vi "Teleop.vi"(10 "Match Info":T1={"Autonomous Elapsed Seconds"=0.0, "TeleOp Elapsed Seconds"=0.0, "Disabled Elapsed Seconds"=0.0, "Visited Autonomous"=FALSE, "Visited TeleOp"=FALSE, "Visited Disabled"=FALSE, "Autonomous Settings"={"Autonomous Style"=enum."Independent", "VI Refnum"=refnum}}, 11 "Call Context":T2) -> ()   [LabVIEW 2023]
doc: "This VI is called for each TeleOp packet received from the DS where the robot is not disabled. It is often used to read from the joysticks and update I/O or to update setpoints for timed control loops. It should complete and return within 20 milliseconds or it may miss DS packets."
uses:
  <vilib>/Rock Robotics/WPI/DriverStation/WPI_DriverStationDerivedRobotMode.ctl
  <vilib>/Rock Robotics/WPI/DriverStation/WPI_DriverStationMatch Info.ctl
  <vilib>/Rock Robotics/WPI/Utilities/WPI_GetSetVariantRefNum.vi
  <vilib>/Rock Robotics/Network Tables/NT Write Boolean Array.vi
  <vilib>/Rock Robotics/Network Tables/NT Write Numeric Array.vi
  <vilib>/Rock Robotics/Network Tables/NT Read Boolean.vi
  <vilib>/Rock Robotics/Network Tables/NT Read Number.vi
  <vilib>/Rock Robotics/WPI/RobotDrive/WPI_RobotDriveMecanumDrive_Cartesian.vi
panel:
  out "Sample Slider 0":dbl(slide) scale=0.0..5.0
  out "Sample Boolean 1":bool
  out "Sample Boolean 0":bool
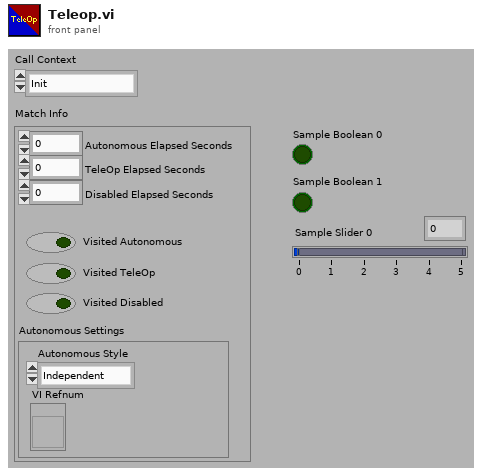
[diagram p1: front panel]
types:
  T1 = typedef "WPI_DriverStationMatch Info.ctl" = cluster{"Autonomous Elapsed Seconds":dbl, "TeleOp Elapsed Seconds":dbl, "Disabled Elapsed Seconds":dbl, "Visited Autonomous":bool, "Visited TeleOp":bool, "Visited Disabled":bool, "Autonomous Settings":cluster{"Autonomous Style":enum16{"Iterative", "Independent"}, "VI Refnum":refnum<vi>}}
  T2 = typedef "WPI_DriverStationDerivedRobotMode.ctl" = enum16{"Init", "Execute", "Stop"}
  T3 = typedef "WPI_JoystickDevRef.ctl" = cluster{"Device":T4}
  T4 = typedef "WPI_JoystickDeviceEnum.ctl" = enum16{"USB 0", "USB 1", "USB 2", "USB 3", "USB 4", "USB 5"}
  T5 = typedef "WPI_MotorControlDeviceRef.ctl" = cluster{"DeviceStatus":errorcluster, "Type":T6, "PWM":cluster{"PWM Channel":T7, "DeadBand":T8}, "CAN":cluster{"Device Number":u8, "SetOutput VI Ref":variant, "GetOutput VI Ref":variant, "Enable VI Ref":variant, "Disable VI Ref":variant, "Data":variant}, "Invert":bool, "DIO PWM":cluster{"PWM \"Enable\" Channel":T7, "DIOChannel":T9, "PWM Rate":dbl}}
  T6 = typedef "WPI_MotorControlType.ctl" = enum16{"PWM", "CAN", "DIO PWM"}
  T7 = typedef "FPGA_DIOPWMChannel.ctl" = enum8{"PWM 0", "PWM 1", "PWM 2", "PWM 3", "PWM 4", "PWM 5", "PWM 6", "PWM 7", "PWM 8", "PWM 9", "PWM MXP 0", "PWM MXP 1", "PWM MXP 2", "PWM MXP 3", "PWM MXP 4", "PWM MXP 5", "PWM MXP 6", "PWM MXP 7", "PWM MXP 8", "PWM MXP 9", "Invalid"}
  T8 = typedef "WPI_PWMDeadband.ctl" = cluster{"Name":string, "maxPositivePwm":i32, "minPositivePwm":i32, "centerPwm":i32, "maxNegativePwm":i32, "minNegativePwm":i32, "angularRange":u16}
  T9 = typedef "FPGA_DIOChannel.ctl" = enum8{"DIO 0", "DIO 1", "DIO 2", "DIO 3", "DIO 4", "DIO 5", "DIO 6", "DIO 7", "DIO 8", "DIO 9", "DIO MXP 0", "DIO MXP 1", "DIO MXP 2", "DIO MXP 3", "DIO MXP 4", "DIO MXP 5", "DIO MXP 6", "DIO MXP 7", "DIO MXP 8", "DIO MXP 9", "DIO MXP 10", "DIO MXP 11", "DIO MXP 12", "DIO MXP 13", "DIO MXP 14", "DIO MXP 15", "SPI Port CS1", "SPI Port CS2", "SPI Port CS3", "SPI Port MISO", "SPI Port MOSI", "Invalid"}
  T10 = typedef "WPI_DigitalInputDevRef.ctl" = cluster{"DevStatus":errorcluster, "DIO Channel":T9}
  T11 = typedef "WPI_RobotDriveDevRef.ctl" = cluster{"DevStatus":errorcluster, "Motors[]":T5[], "Square Inputs":bool, "Max Output":dbl}
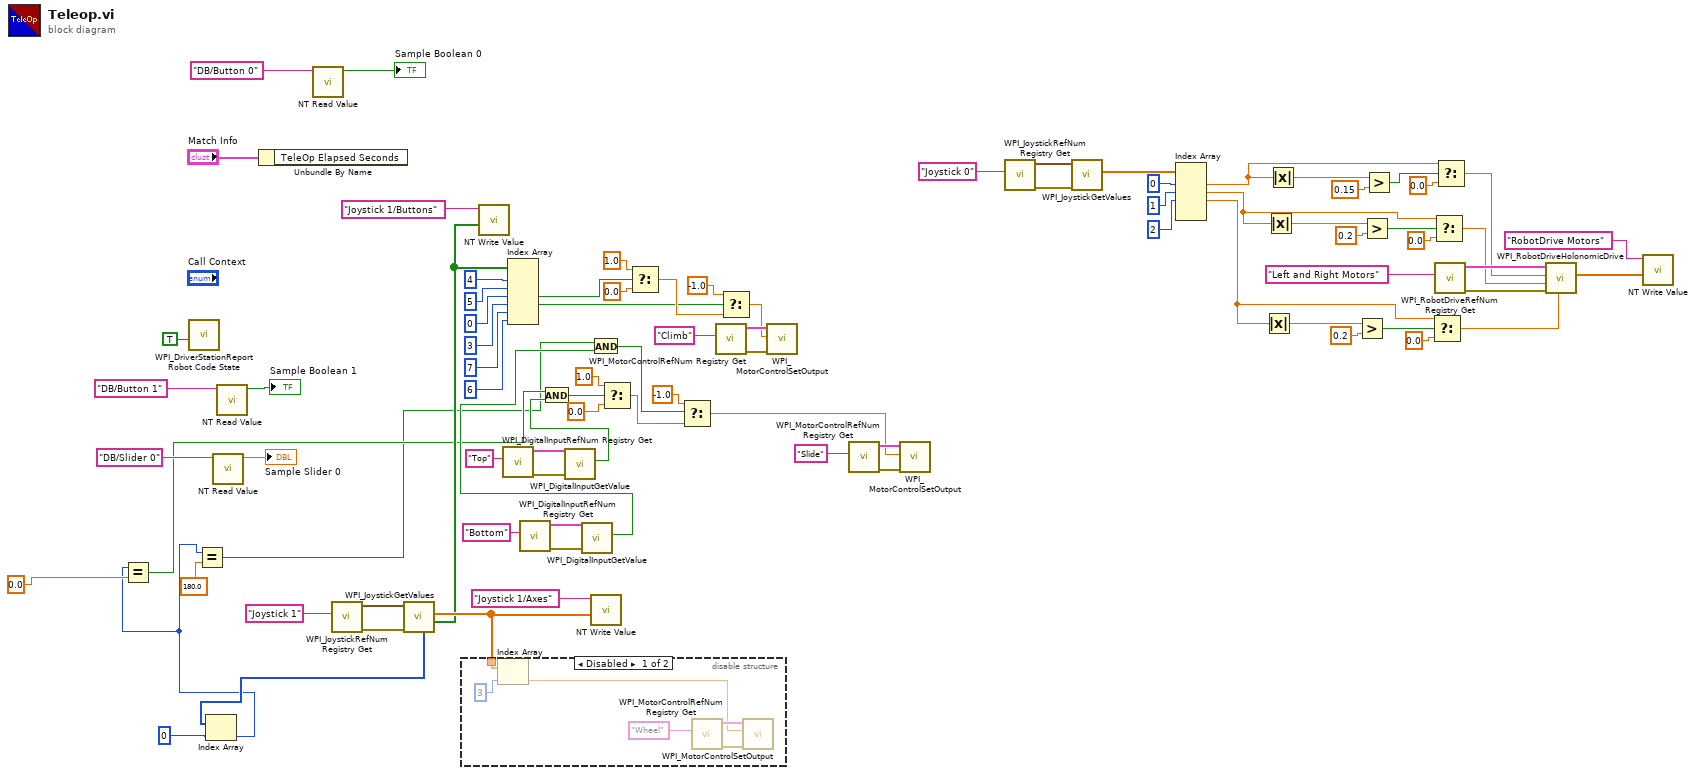
[diagram p0: block diagram]
diagram:
  n1 = call <vilib>:"WPI_DriverStationReport Robot Code State.vi"("TeleOp"=TRUE ("Autonomous")) -> ()  [unwired: 10 in, 1 out]
  n2 = call-poly <vilib>:"NT Read Value.vi"("name"="DB/Slider 0" ("refnum name")) -> ("value"=→"Sample Slider 0":dbl)  [unwired: 8 in, 2 out]
  n3 = call-poly <vilib>:"NT Read Value.vi"("name"="DB/Button 1" ("refnum name")) -> ("value"=→"Sample Boolean 1":bool)  [unwired: 8 in, 2 out]
  n4 = Unbundle By Name("Match Info") -> ()  [unwired: 1 out]
  n5 = call-poly <vilib>:"NT Read Value.vi"("name"="DB/Button 0" ("refnum name")) -> ("value"=→"Sample Boolean 0":bool)  [unwired: 8 in, 2 out]
  n6 = call <vilib>:"WPI_JoystickRefNum Registry Get.vi"("refnum name"="Joystick 1") -> ("error out"=w69:errorcluster, "JoystickDevRef"=w82:T3)  [unwired: 1 in, 8 out]
  n7 = call <vilib>:"WPI_JoystickGetValues.vi"("error in (no error)"=w69, "JoystickDevRef"=w82) -> ("Buttons"=w23:bool[], "Axes"=w78:dbl[], "POVs"=w9:i16[])  [unwired: 5 in, 2 out]
  n8 = Index Array(array=w9, index=0) -> (element=w6:i16)
  n9 = Equal?(x=w6, y=0.0 ("Output")) -> (x = y?=w11:bool)
  n10 = Equal?(x=w6, y=180.0 ("Output")) -> (x = y?=w10:bool)
  n11 = disable-structure shown="Disabled" {
    disable-tunnel: w78 -> [w92 _]
    frame Disabled {
      n12 = Index Array(array=w92, index=3) -> (element=w87:dbl)
      n13 = call <vilib>:"WPI_MotorControlRefNum Registry Get.vi"("refnum name"="Wheel") -> ("error out"=w89:errorcluster, "MotorControlDevRef"=w90:T5)  [unwired: 9 in]
      n14 = call <vilib>:"WPI_MotorControlSetOutput.vi"("error in (no error)"=w89, "Output"=w87, "MotorControlDevRef"=w90) -> ()  [unwired: 6 in, 3 out]
    }
    frame Enabled {
    }
  }
  n15 = call-poly <vilib>:"NT Write Value.vi"("value"=w23, "name"="Joystick 1/Buttons" ("Name")) -> ()  [unwired: 9 in, 1 out]
  n16 = call <vilib>:"WPI_DigitalInputRefNum Registry Get.vi"("refnum name"="Top") -> ("error out"=w18:errorcluster, "DigitalInputDevRef"=w17:T10)  [unwired: 9 in]
  n17 = Index Array(array=w23, index #1=4 ("index"), index #2=5 ("index"), index #3=0 ("index"), index #4=3 ("index"), index #5=7 ("index"), index #6=6 ("index")) -> (element #3=w63:bool, element #4=w41:bool)  [unwired: 4 out]
  n18 = call <vilib>:"WPI_DigitalInputRefNum Registry Get.vi"("refnum name"="Bottom") -> ("error out"=w21:errorcluster, "DigitalInputDevRef"=w22:T10)  [unwired: 9 in]
  n19 = call <vilib>:"WPI_DigitalInputGetValue.vi"("error in (no error)"=w18, "DigitalInputDevRef"=w17) -> ("Value"=w16:bool)  [unwired: 7 in, 2 out]
  n20 = And(x=w11, y=w16) -> (x .and. y?=w7:bool)
  n21 = call <vilib>:"WPI_DigitalInputGetValue.vi"("error in (no error)"=w21, "DigitalInputDevRef"=w22) -> ("Value"=w14:bool)  [unwired: 7 in, 2 out]
  n22 = And(x=w10, y=w14) -> (x .and. y?=w15:bool)
  n23 = call-poly <vilib>:"NT Write Value.vi"("value"=w78, "name"="Joystick 1/Axes" ("Name")) -> ()  [unwired: 9 in, 1 out]
  n24 = Select(t=1.0 ("Output"), s=w7, f=0.0 ("Output")) -> (s? t:f=w40:dbl)
  n25 = Select(t=1.0 ("Output"), s=w63, f=0.0 ("Output")) -> (s? t:f=w42:dbl)
  n26 = Select(t=-1.0 ("Output"), s=w15, f=w40) -> (s? t:f=w2:dbl)
  n27 = call <vilib>:"WPI_MotorControlRefNum Registry Get.vi"("refnum name"="Climb") -> ("error out"=w60:errorcluster, "MotorControlDevRef"=w61:T5)  [unwired: 9 in]
  n28 = Select(t=-1.0 ("Output"), s=w41, f=w42) -> (s? t:f=w1:dbl)
  n29 = call <vilib>:"WPI_MotorControlSetOutput.vi"("error in (no error)"=w60, "Output"=w1, "MotorControlDevRef"=w61) -> ()  [unwired: 6 in, 3 out]
  n30 = call <vilib>:"WPI_MotorControlRefNum Registry Get.vi"("refnum name"="Slide") -> ("error out"=w3:errorcluster, "MotorControlDevRef"=w4:T5)  [unwired: 9 in]
  n31 = call <vilib>:"WPI_MotorControlSetOutput.vi"("error in (no error)"=w3, "Output"=w2, "MotorControlDevRef"=w4) -> ()  [unwired: 6 in, 3 out]
  n32 = call <vilib>:"WPI_JoystickRefNum Registry Get.vi"("refnum name"="Joystick 0") -> ("error out"=w31:errorcluster, "JoystickDevRef"=w26:T3)  [unwired: 1 in, 8 out]
  n33 = call <vilib>:"WPI_JoystickGetValues.vi"("error in (no error)"=w31, "JoystickDevRef"=w26) -> ("Axes"=w34:dbl[])  [unwired: 5 in, 4 out]
  n34 = Index Array(array=w34, index #1=0 ("index"), index #2=1 ("index"), index #3=2 ("index")) -> (element #1=w29:dbl, element #2=w28:dbl, element #3=w27:dbl)  [unwired: 2 in, 2 out]
  n35 = Absolute Value(x=w27) -> (abs(x)=w48:dbl)
  n36 = Absolute Value(x=w28) -> (abs(x)=w52:dbl)
  n37 = Absolute Value(x=w29) -> (abs(x)=w58:dbl)
  n38 = Greater?(x=w48, y=0.2) -> (0:w46:bool)
  n39 = Greater?(x=w52, y=0.2) -> (0:w54:bool)
  n40 = Greater?(x=w58, y=0.15) -> (0:w56:bool)
  n41 = Select(t=w27, s=w46, f=0.0) -> (s? t:f=w45:dbl)
  n42 = Select(t=w28, s=w54, f=0.0) -> (s? t:f=w50:dbl)
  n43 = call <vilib>:"WPI_RobotDriveRefNum Registry Get.vi"("refnum name"="Left and Right Motors") -> ("error out"=w68:errorcluster, "RobotDriveDevRef"=w84:T11)  [unwired: 1 in, 8 out]
  n44 = Select(t=w29, s=w56, f=0.0) -> (s? t:f=w55:dbl)
  n45 = call-poly <vilib>:"WPI_RobotDriveHolonomicDrive.vi"("Rotation"=w45, "error in (no error)"=w68, "Y"=w50, "X"=w55, "RobotDriveDevRef"=w84) -> ("Motor Values"=w71:dbl[])  [unwired: 4 in, 2 out]
  n46 = call-poly <vilib>:"NT Write Value.vi"("value"=w71, "name"="RobotDrive Motors" ("Name")) -> ()  [unwired: 9 in, 1 out]
